vi "Test Helper Loop No Time Out Stopping if Error Loop Finished.vi"(8 "error in (no error)":errorcluster, 11 "Helper Loop Test In":refnum<class "Helper Loop Test.lvclass">) -> (0 "error out":errorcluster, 3 "Helper Loop Test Out":refnum<class "Helper Loop Test.lvclass">)   [LabVIEW 2020, in "Helper Loop Test.lvclass"]
uses:
  Helper Loop Test.lvclass
  C:/Program Files (x86)/National Instruments/LabVIEW 2020/vi.lib/Asteme/LUnit/Test Case.lvclass
  Mock Process/Mock Process.lvclass
  C:/Users/anton/Documents/GitHub/Triarc-Framework/source/Framework/Process/Process.lvclass
  <vilib>/Asteme/LUnit/Test Case.lvclass/Test Case.ctl
  <vilib>/Asteme/LUnit/LUnit Assertion Result.lvclass/LUnit Assertion Result.ctl
  Framework/Process/Process.lvclass/Process.ctl
  <vilib>/Asteme/LUnit/Palette/Pass If.vi
  <vilib>/Asteme/LUnit/Set Assertion Type.vi
  Framework/Process/Private/SubVIs/Wait for finish.vi
  Framework/Process/Protected/Messaging/Enqueue Message.vi
  Framework/Process/Private/SubVIs/Set Lifecycle State.vi
  Framework/Process/Public/Lifecycle/Get Lifecycle State.vi
  <vilib>/Asteme/LUnit/Palette/Fail.vi
  <vilib>/Asteme/LUnit/Palette/Pass.vi
  <vilib>/Asteme/LUnit/LUnit Write Assertion Type.vi
  <vilib>/Utility/error.llb/Clear Errors.vi
  <vilib>/Asteme/LUnit/Add test result.vi
  <vilib>/Asteme/LUnit/LUnit Write Passed.vi
  <vilib>/Asteme/LUnit/LUnit Get Test Case.vi
  <vilib>/Asteme/LUnit/Assertion Result/LUnit Get Test Name.vi
  <vilib>/Asteme/LUnit/LUnit Write Message.vi
  <vilib>/Asteme/LUnit/LUnit Write Description.vi
  <vilib>/Asteme/LUnit/Read Test Case Name.vi
  <vilib>/Utility/error.llb/Error Cluster From Error Code.vi
  <vilib>/Asteme/LUnit/LUnit Assertion Result.lvclass
  Framework/Process/Process.lvclass
  <vilib>/Asteme/LUnit/Test Case.lvclass
panel:
  out "timed out?":bool
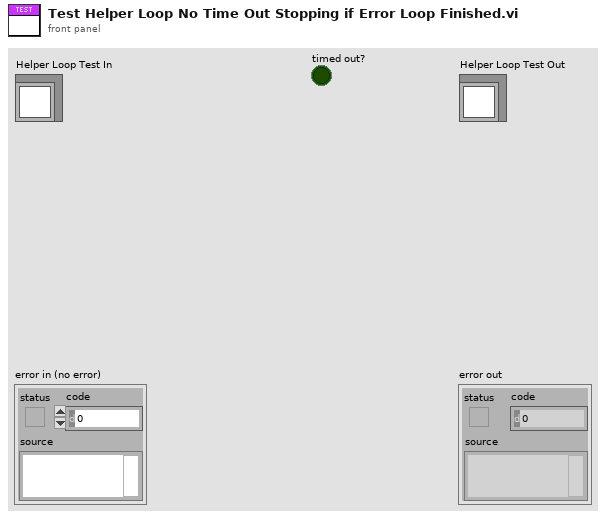
[diagram p1: front panel]
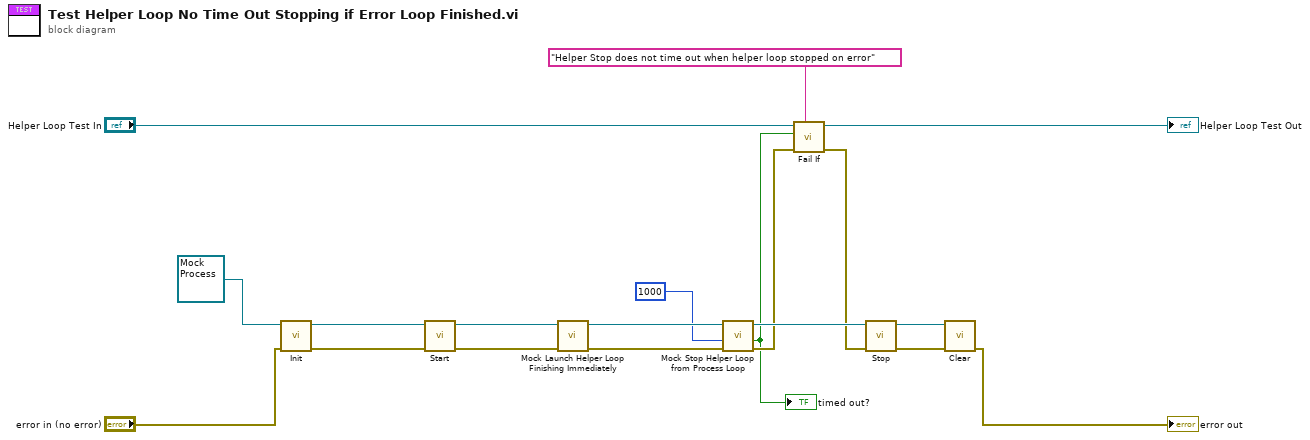
[diagram p0: block diagram]
diagram:
  n1 = call-dynamic "Init.vi"("error in (no error)"="error in (no error)", "Mock Process In"=refnum<class "Mock Process.lvclass"> refnum) -> ("error out"=w18:errorcluster, "Mock Process Out"=w19:refnum<class "Mock Process.lvclass">)  [unwired: 8 in]
  n2 = call "Start.vi"("error in (no error)"=w18, "Process In"=w19) -> ("error out"=w16:errorcluster, "Process Out"=w17:refnum<class "Mock Process.lvclass">)  [unwired: 8 in]
  n3 = call "Mock Launch Helper Loop Finishing Immediately.vi"("error in (no error)"=w16, "Mock Process in"=w17) -> ("error out"=w8:errorcluster, "Mock Process out"=w15:refnum<class "Mock Process.lvclass">)  [unwired: 8 in]
  n4 = call "Mock Stop Helper Loop from Process Loop.vi"("error in (no error)"=w8, "timeout in ms (-1)"=1000, "Mock Process in"=w15) -> ("error out"=w13:errorcluster, "timed out?"=w2:bool, "Mock Process out"=w14:refnum<class "Mock Process.lvclass">)  [unwired: 6 in]
  "timed out?" <- w2
  n5 = call <vilib>:"Fail If.vi"("Description"="Helper Stop does not time out when helper loop stopped on error", "error in (no error)"=w13, "Fail?"=w2, "Test Case In"="Helper Loop Test In") -> ("error out"=w5:errorcluster, "Test Case Out"=→"Helper Loop Test Out":refnum<class "Helper Loop Test.lvclass">)  [unwired: 6 in]
  n6 = call "Stop.vi"("error in (no error)"=w5, "Process In"=w14) -> ("error out"=w12:errorcluster, "Process Out"=w1:refnum<class "Mock Process.lvclass">)  [unwired: 7 in, 1 out]
  n7 = call-dynamic "Clear.vi"("error in (no error)"=w12, "Mock Process In"=w1) -> ("error out"=→"error out":errorcluster)  [unwired: 9 in]
